vi "Ethernet Reader.vi"(0 "IP":string="127.0.0.1", 1 "포트":u16=50, 3 "에러 입력(에러 없음)":errorcluster) -> (6 "Axis":string, 9 "에러 출력":errorcluster={"status"=TRUE, "code"=56, "source"="Ethernet Reader.vi 안에 UDP 읽기"})   [LabVIEW 2013]
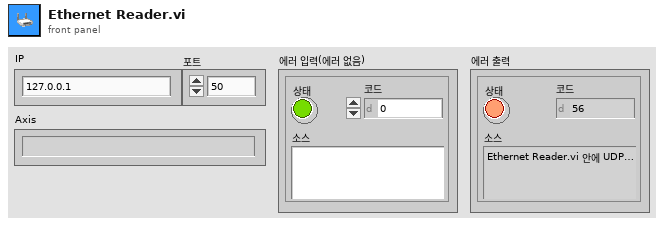
[diagram p1: front panel]
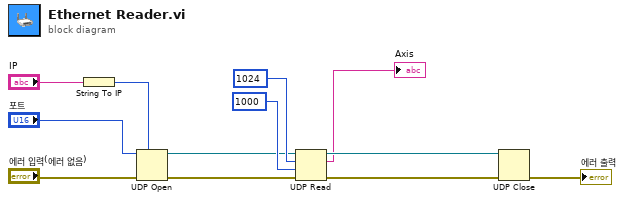
[diagram p0: block diagram]
diagram:
  n1 = String To IP(1:"IP") -> (0:w6:u32)
  n2 = UDP Open(7:w6, 8:"에러 입력(에러 없음)", 11:"포트") -> (port=w2:refnum<k16>, 0:w3:errorcluster)  [unwired: 2 in, 1 out]
  n3 = UDP Read(connection ID=w2, max size (548)=1024 ("최대 크기(548)"), timeout ms (25000)=1000 ("타임아웃 ms (25000)"), 8:w3) -> (data out=→"Axis":string, error out=w10:errorcluster, 3:w9:refnum<k16>)  [unwired: 2 out]
  n4 = UDP Close(connection ID=w9, 8:w10) -> (error out=→"에러 출력":errorcluster)  [unwired: 1 out]
